vi "ROS for LabVIEW Software.vi"   [LabVIEW 2015]
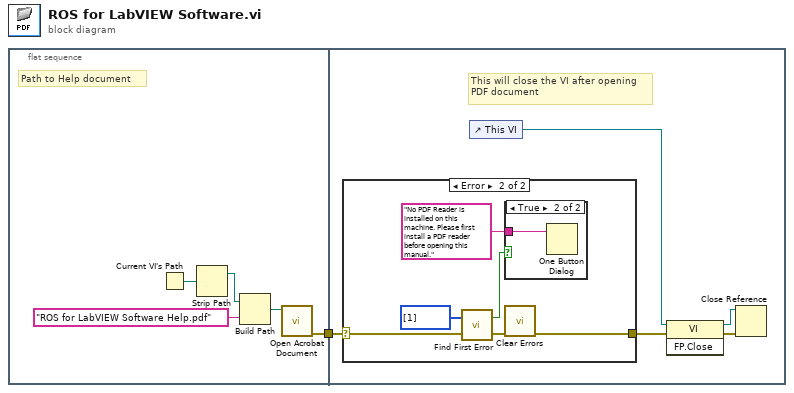
[diagram p0: block diagram]
diagram:
  n1 = flat-sequence {
    tunnel: [w6] -> w1
    tunnel: w1 -> [w8]
    frame #0 {
      # "Path to Help document"
      n2 = Current VI's Path() -> (path=w5:path)
      n3 = Strip Path(path=w5) -> (stripped path=w4:path)  [unwired: 1 out]
      n4 = Build Path(base path=w4, name or relative path="ROS for LabVIEW Software Help.pdf") -> (appended path=w3:path)
      n5 = call "Open Acrobat Document.vi"("acrobat document"=w3) -> ("error out"=w6:errorcluster)  [unwired: 6 in]
    }
    frame #1 {
      # "This will close the VI after opening\nPDF document"
      n6 = case shown="Error" w8 {
        selector: w8 -> [w12 w18]
        tunnel: [w12 w15] -> w7
        frame No Error {
        }
        frame Error {
          n7 = call "Find First Error.vi"("error in (no error)"=w18, "error codes"=i32[] [1]) -> ("error out"=w16:errorcluster, "error?"=w14:bool)  [unwired: 2 in]
          n8 = case shown="True" w14 {
            tunnel: "No PDF Reader is installed on this machine. Please first install a PDF reader before opening this manual." -> [_ w19]
            frame False {
            }
            frame True {
              n9 = One Button Dialog(message=w19) -> ()  [unwired: 1 in, 1 out]
            }
          }
          n10 = call "Clear Errors.vi"("error in (no error)"=w16) -> ("error out"=w15:errorcluster)  [unwired: 5 in, 1 out]
        }
      }
      n11 = control-ref of="This VI"() -> (w9:refnum<vi>)
      n12 = invoke class="VI" method="FP.Close"(reference=w9, error in=w7) -> (reference out=w11:refnum<vi>, error out=w10:errorcluster)  [unwired: 1 in, 1 out]
      n13 = Close Reference(reference=w11, error in (no error)=w10) -> ()  [unwired: 1 out]
    }
  }
